vi "Update Values Buffer.vi"(7 "byte order (little-endian)":T1=enum."little-endian", 8 "error in":errorcluster, 9 "buffer data":T2={"decimation"=0, "avg bandwidth"=0.0, "channels"=[], "byte order"=enum."little-endian", "buffer descriptor"={"buffer type"=enum."Engine", "plugin id"=0, "group id"=0, "transfer id"=0, "offset"=0, "length"=0}, "values channels"={"index"=0, "count"=0, "engine offset"=0}, "select start offset"=18446744073709551615, "select end offset"=0, "channel index"=-1} {"channels"."configuration"."string offset" format="%d bytes"; "avg bandwidth" format="%.0g bytes"}, 10 "buffer in":u8[](array[numeric]), 11 "values buffer in":u8[](array[numeric])) -> (0 "error out":errorcluster, 2 "buffer out":u8[](array[numeric]), 3 "values buffer out":u8[](array[numeric]))   [LabVIEW 2020, in "DSF Core.lvlib"]
uses:
  DSF Core.lvlib
  Classes/Framework/Framework.lvclass
  Typedefs/DSF Byte Order.ctl
  Typedefs/DSF Data Type.ctl
  Typedefs/DSF Settings Info.ctl
  Typedefs/DSF Buffer Type.ctl
  Classes/Thread/Data Server/DSF Buffer Subset Descriptor.ctl
  Values Channels.ctl
  Buffer Reader/Buffer Data.ctl
  Typedefs/Core Channel Configuration.ctl
  Classes/Configuration/Core/Channel/Channel Configuration.lvclass
  Classes/Configuration/Core/Transfer/Channel Configuration.ctl
  Classes/Configuration/Core/Transfer/Transfer Configuration.lvclass
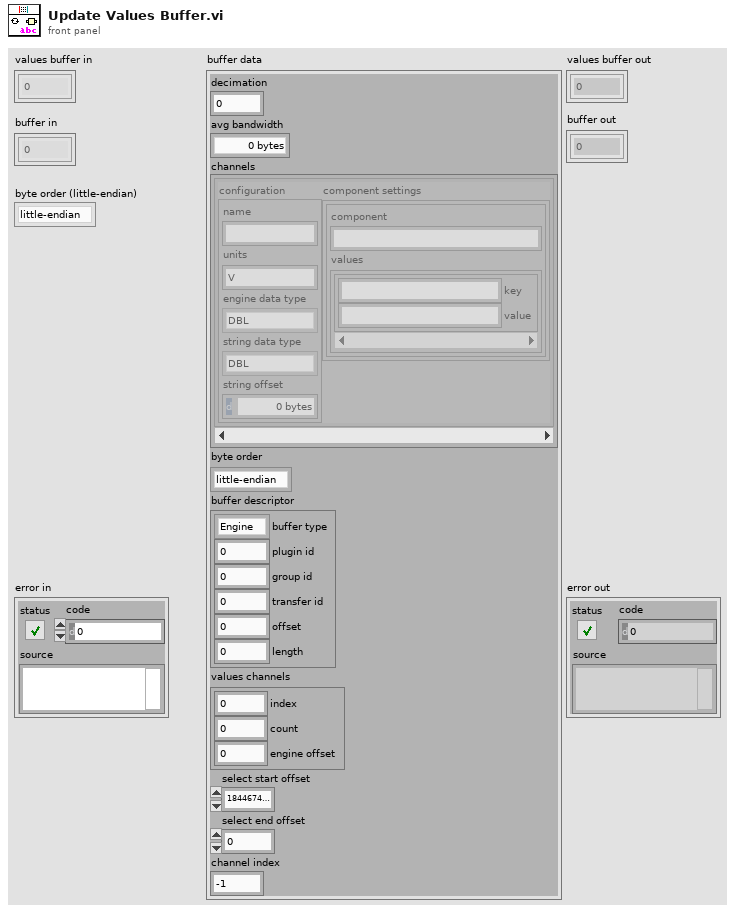
[diagram p1: front panel]
types:
  T1 = typedef "DSF Core.lvlib/DSF Byte Order.ctl" = enum8{"big-endian", "little-endian"}
  T2 = typedef "DSF Core.lvlib/Buffer Data.ctl" = cluster{"decimation":u64, "avg bandwidth":dbl, "channels":T3[], "byte order":T1, "buffer descriptor":T7, "values channels":T9, "select start offset":u64, "select end offset":u64, "channel index":i32}
  T3 = typedef "DSF Core.lvlib/Transfer Configuration.lvclass/Channel Configuration.ctl" = cluster{"configuration":T4, "component settings":T6[]}
  T4 = typedef "DSF Core.lvlib/Channel Configuration.lvclass/Core Channel Configuration.ctl" = cluster{"name":string, "units":string, "engine data type":T5, "string data type":T5, "string offset":u64}
  T5 = typedef "DSF Core.lvlib/DSF Data Type.ctl" = enum8{"Bool", "SGL", "DBL", "I8", "I16", "I32", "I64", "U8", "U16", "U32", "U64"}
  T6 = typedef "DSF Core.lvlib/DSF Settings Info.ctl" = cluster{"component":string, "values":cluster{"key":string, "value":string}[]}
  T7 = typedef "DSF Core.lvlib/DSF Buffer Subset Descriptor.ctl" = cluster{"buffer type":T8, "plugin id":i32, "group id":i32, "transfer id":i32, "offset":u64, "length":i64}
  T8 = typedef "DSF Core.lvlib/DSF Buffer Type.ctl" = enum16{"Engine", "String"}
  T9 = typedef "DSF Core.lvlib/Values Channels.ctl" = cluster{"index":i32, "count":i32, "engine offset":u64}
  T10 = enum16{"big-endian, network order", "native, host order", "little-endian"}
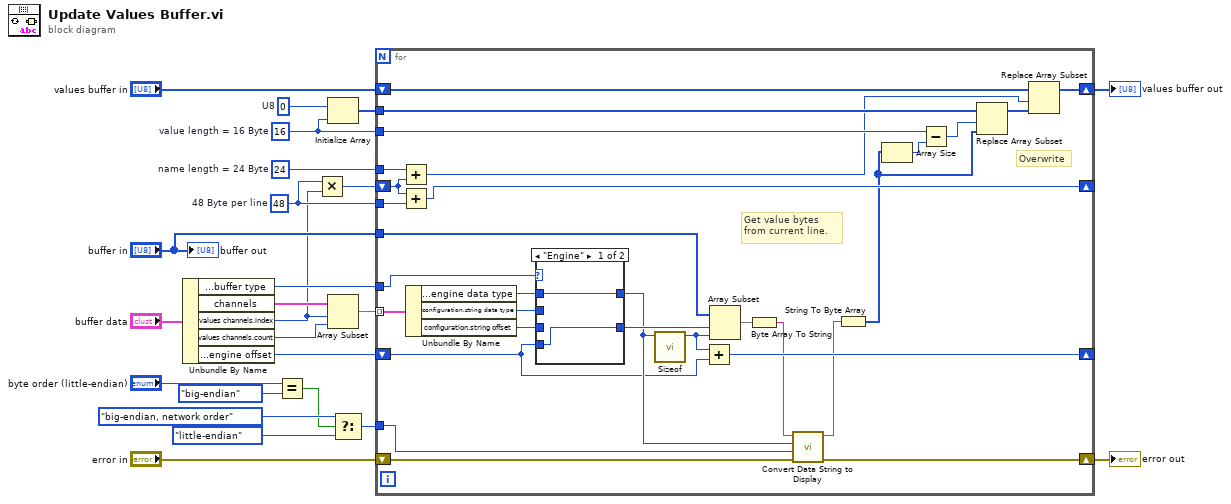
[diagram p0: block diagram]
diagram:
  w3 = u8 0  # U8
  w1 = 16  # value length = 16 Byte
  w4 = 24  # name length = 24 Byte
  w9 = 48  # 48 Byte per line
  n1 = Unbundle By Name("buffer data") -> ("buffer descriptor.buffer type"=w22:T8, "channels"=w21:T3[], "values channels.index"=w7:i32, "values channels.count"=w6:i32, "values channels.engine offset"=w5:u64)
  n2 = Equal?(x="byte order (little-endian)", y=DSF_Byte_Order."big-endian") -> (x = y?=w12:bool)
  n3 = Multiply(x=w9, y=w7) -> (x*y=w10:i32)
  n4 = Initialize Array(w3, w1) -> (w2:u8[])
  n5 = Array Subset(array=w21, index=w7, length=w6) -> (w24:T3[])
  n6 = Select(t=T10."big-endian, network order" ("byte order (0:big-endian, network order)"), s=w12, f=T10."little-endian") -> (s? t:f=w17:T10)
  n7 = for {
    shift-right: [w36] -> w14
    shift-left: "error in" -> [w54]
    tunnel: w24 -> [w53] mode=indexing
    tunnel: w22 -> [w47]
    shift-right: [w48] -> _
    shift-left: w5 -> [w25]
    tunnel: w17 -> [w44]
    shift-right: [w45] -> w15
    shift-left: "values buffer in" -> [w46]
    tunnel: "buffer in" -> [w43]
    shift-right: [w37] -> _
    shift-left: w10 -> [w38]
    tunnel: w9 -> [w39]
    tunnel: w4 -> [w29]
    tunnel: w2 -> [w28]
    tunnel: w1 -> [w27]
    # "Overwrite"
    # "Get value bytes from current line."
    n8 = Add(x=w29, y=w38) -> (x+y=w26:i32)
    n9 = Add(x=w38, y=w39) -> (x+y=w37:i32)
    n10 = Unbundle By Name(w53) -> ("configuration.engine data type"=w50:T5, "configuration.string data type"=w51:T5, "configuration.string offset"=w52:u64)
    n11 = case shown="\"Engine\"" w47 {
      tunnel: w52 -> [_ w58]
      tunnel: [w55 w58] -> w35
      tunnel: w51 -> [_ w57]
      tunnel: w50 -> [w56 _]
      tunnel: w25 -> [w55 _]
      tunnel: [w56 w57] -> w30
      frame "Engine" {
      }
      frame "String" {
      }
    }
    n12 = call "Sizeof.vi"("data type"=w30) -> ("size in bytes"=w49:u64)  [unwired: 9 in, 1 out]
    n13 = Add(x=w49, y=w25) -> (x+y=w48:u64)
    n14 = Array Subset(array=w43, index=w35, length=w49) -> (w34:u8[])
    n15 = Byte Array To String(unsigned byte array=w34) -> (string=w31:string)
    n16 = call "Convert Data String to Display.vi"("error in"=w54, "endianness (little-endian)"=w44, "string data type"=w30, "data string"=w31) -> ("error out"=w36:errorcluster, "display string"=w32:string)  [unwired: 6 in]
    n17 = String To Byte Array(string=w32) -> (unsigned byte array=w33:u8[])
    n18 = Array Size(array=w33) -> (size(s)=w42:i32)
    n19 = Subtract(x=w27, y=w42) -> (x-y=w41:i32)
    n20 = Replace Array Subset(array=w28, new element=w33, index=w41) -> (w40:u8[])
    n21 = Replace Array Subset(array=w46, new element=w40, index=w26) -> (w45:u8[])
  }
  "values buffer out" <- w15
  "error out" <- w14
  "buffer out" <- "buffer in"
